vi "Write DirectOrKickoff.vi"(8 "error in (no error)":errorcluster, 10 "DirectOrKickoff":bool, 11 "Ally in":refnum<class "Ally.lvclass">) -> (0 "error out":errorcluster, 3 "Ally out":refnum<class "Ally.lvclass">)   [LabVIEW 2023, in "Ally.lvclass"]
uses:
  Ally.lvclass
  Ally.lvclass/Ally.ctl
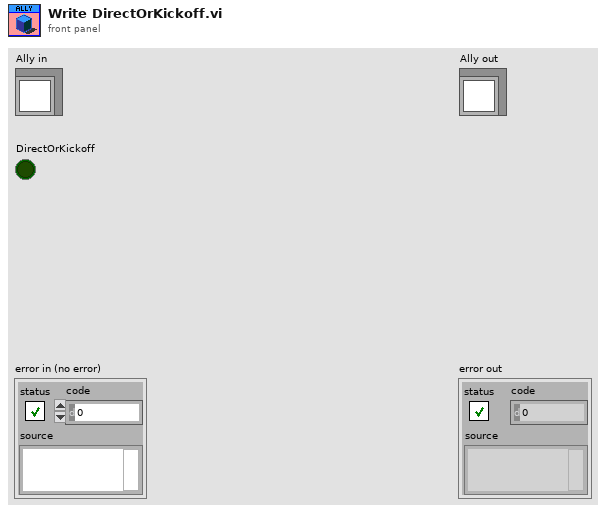
[diagram p1: front panel]
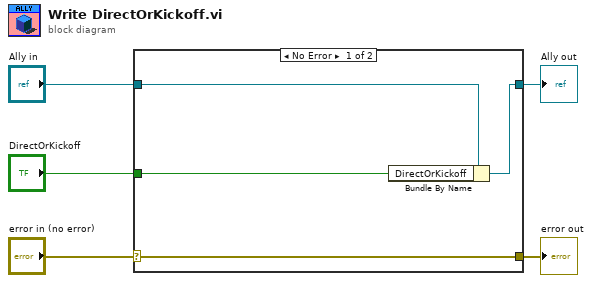
[diagram p0: block diagram]
diagram:
  n1 = case shown="No Error" "error in (no error)" {
    selector: "error in (no error)" -> [w9 w10]
    tunnel: [w9 w10] -> w4
    tunnel: [w7 w11] -> w2
    tunnel: "Ally in" -> [w8 w11]
    tunnel: "DirectOrKickoff" -> [w6 _]
    frame No Error {
      n2 = Bundle By Name(cluster=w8, "DirectOrKickoff"=w6) -> (w7:refnum<class "Ally.lvclass">)
    }
    frame Error {
    }
  }
  "error out" <- w4
  "Ally out" <- w2
